vi "controllerPIP.vi"(11 "error in (no error)":errorcluster) -> (4 "FIXTURE_SETUP-1":string, 6 "POWER_UP-5, 6":string, 8 "RESISTANCE-15":string, 10 "INCLINE-14":string, 15 "error out":errorcluster)   [LabVIEW 2018]
uses:
  Global_1259.vi
panel:
  out "MTA":bool
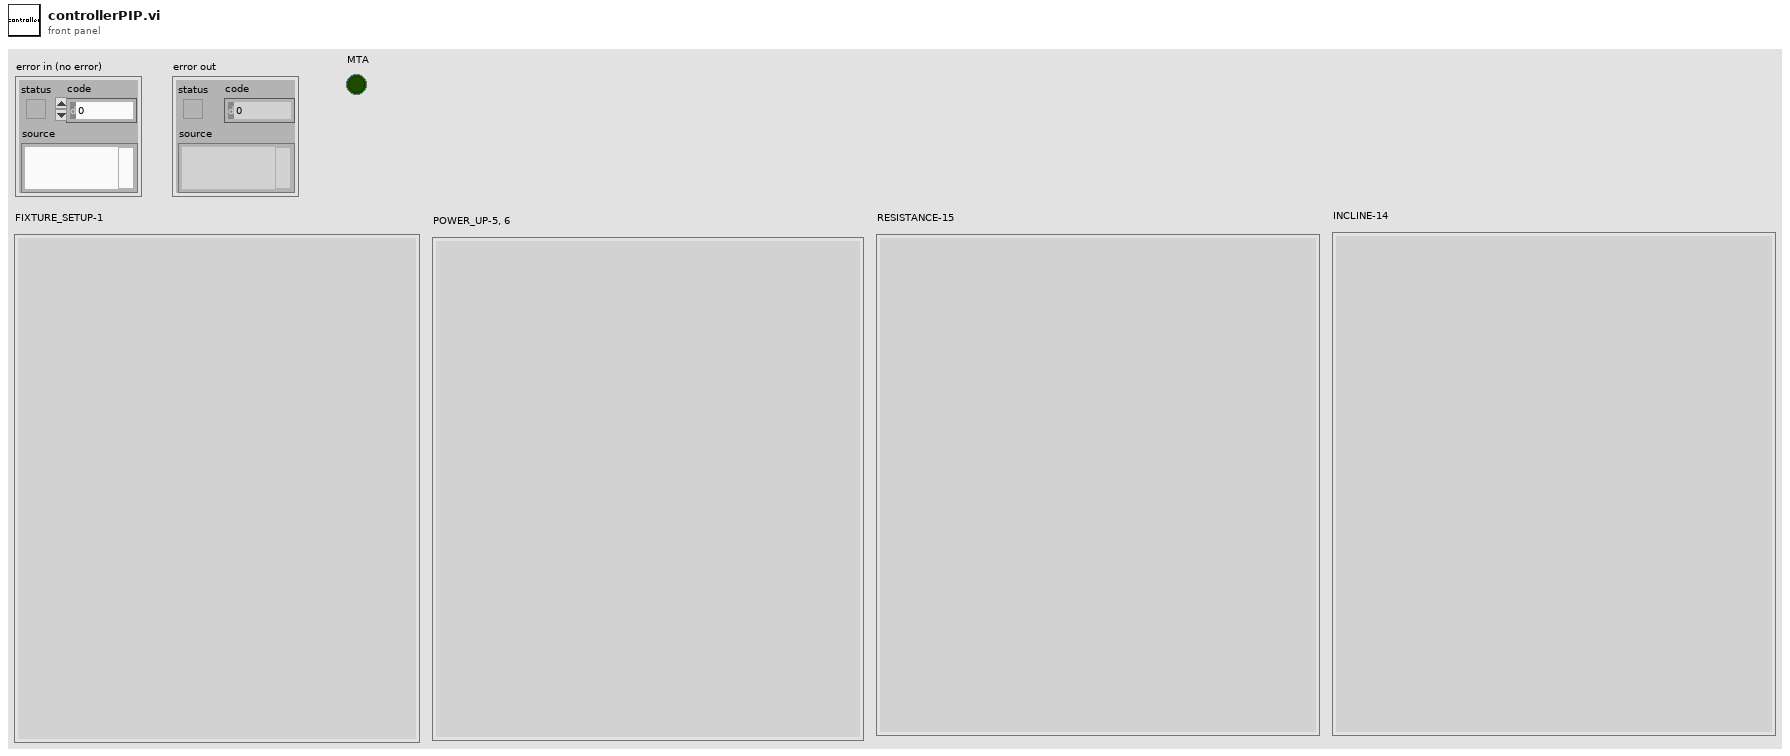
[diagram p1: front panel]
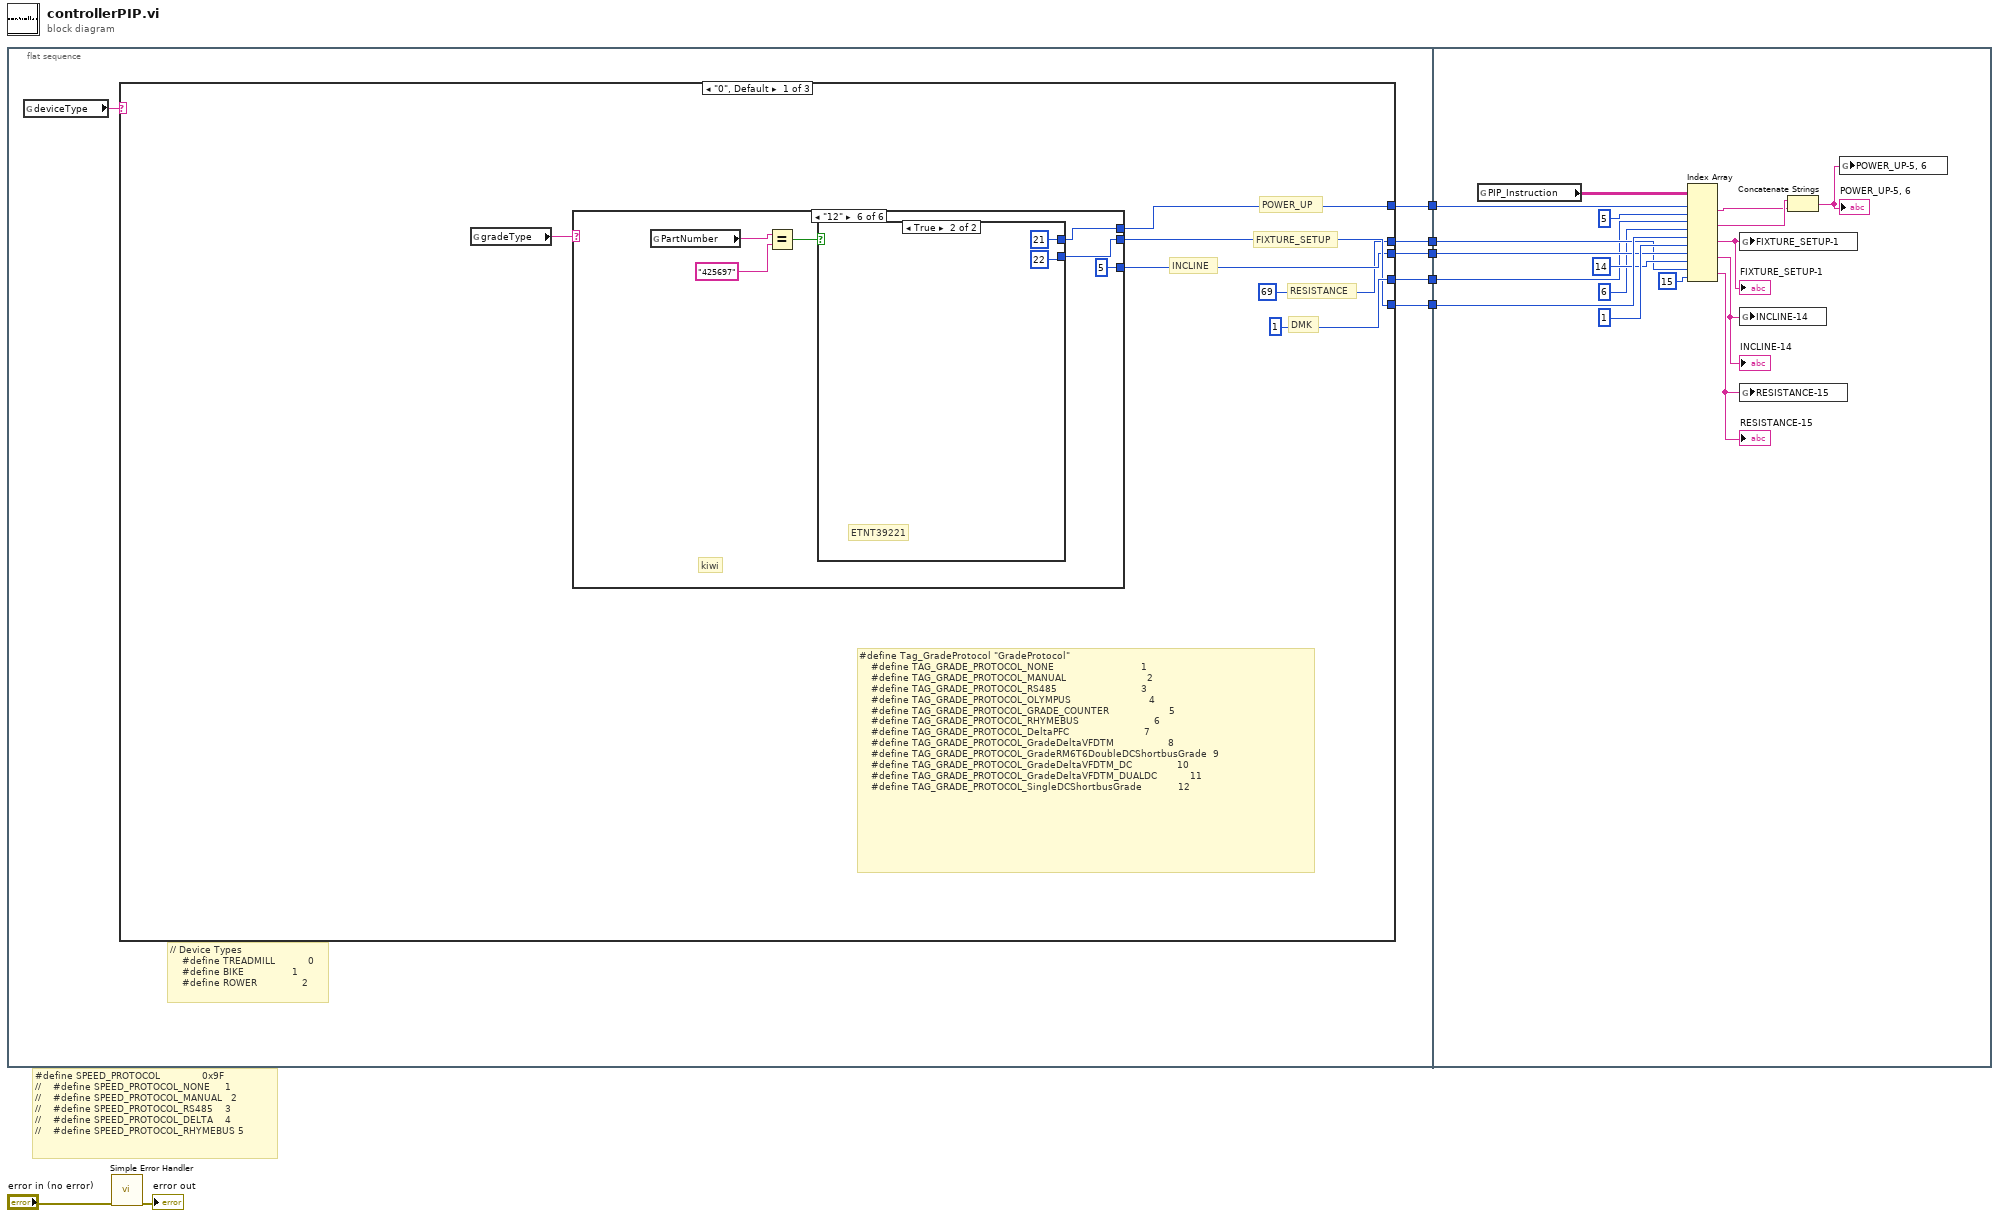
[diagram p0: block diagram]
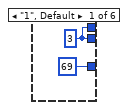
[diagram p2: hidden frame]
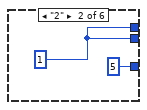
[diagram p3: hidden frame]
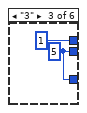
[diagram p4: hidden frame]
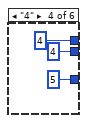
[diagram p5: hidden frame]
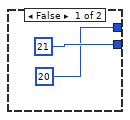
[diagram p7: hidden frame]
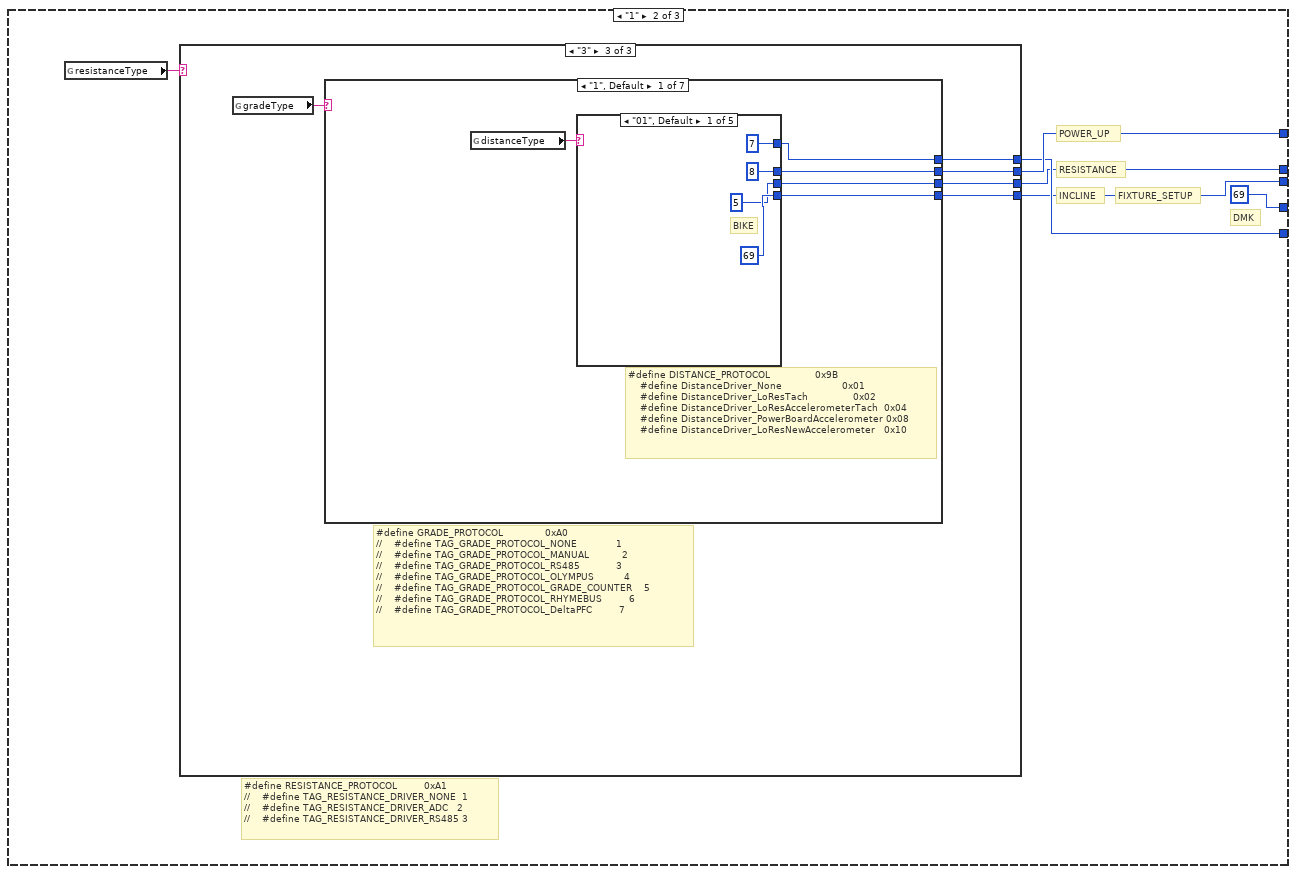
[diagram p8: hidden frame]
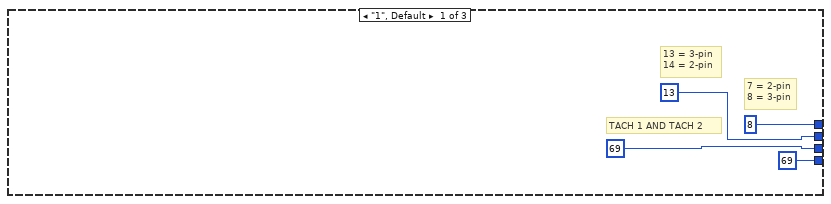
[diagram p9: hidden frame]
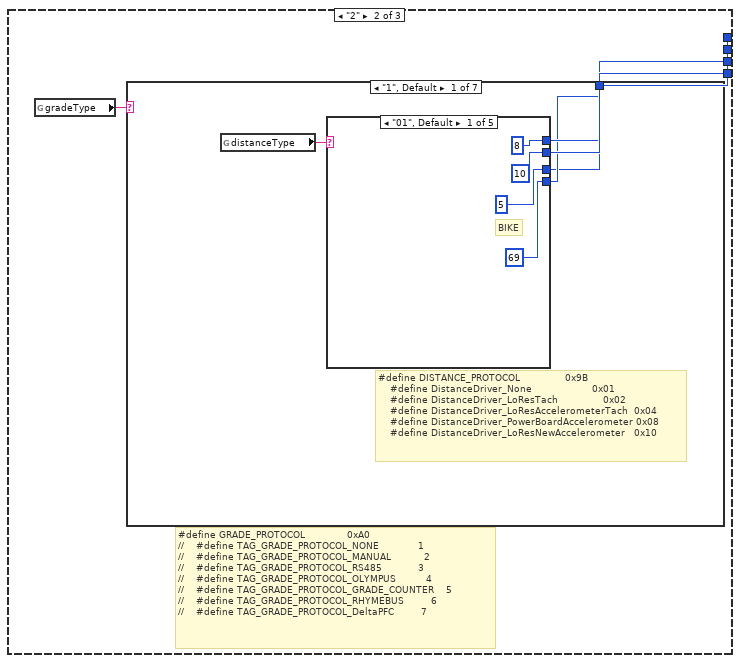
[diagram p10: hidden frame]
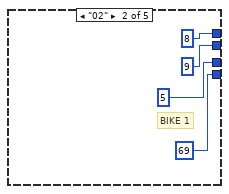
[diagram p11: hidden frame]
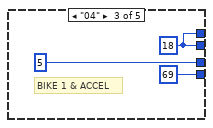
[diagram p12: hidden frame]
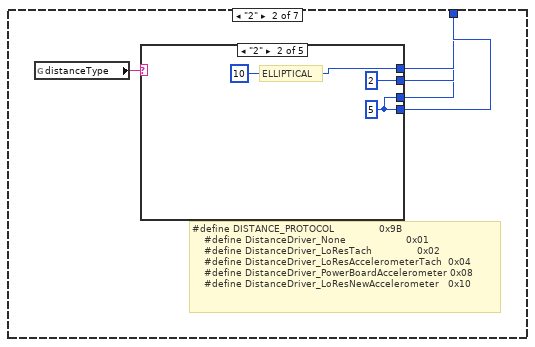
[diagram p15: hidden frame]
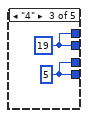
[diagram p17: hidden frame]
diagram:
  # "#define SPEED_PROTOCOL              0x9F\n//    #define SPEED_PROTOCOL_NONE     1\n//    #define SPEED_PROTOCOL_MANUAL   2\n//    #define SPEED_PROTOCOL_RS485    3\n//    #define SPEED_PROTOCOL_DELTA    4\n//    #define SPEED_PROTOCOL_RHYMEBUS 5"
  n1 = flat-sequence {
    tunnel: [w12] -> w7
    tunnel: [w11] -> w6
    tunnel: [w10] -> w5
    tunnel: [w9] -> w2
    tunnel: [w8] -> w1
    tunnel: w7 -> [w161]
    tunnel: w6 -> [w147]
    tunnel: w5 -> [w151]
    tunnel: w2 -> [w158]
    tunnel: w1 -> [w155]
    frame #0 {
      # "// Device Types\n    #define TREADMILL           0\n    #define BIKE                1\n    #define ROWER               2"
      n2 = global read "Global_1259.vi" "deviceType"() -> (w13:string)
      n3 = case shown="\"0\", Default" w13 {
        tunnel: [w17 w42 w116] -> w12
        tunnel: [1 69 w117] -> w11
        tunnel: [w14 w43 w114] -> w10
        tunnel: [w16 w41 w117] -> w9
        tunnel: [69 w40 w115] -> w8
        frame "0", Default {
          # "POWER_UP"
          # "RESISTANCE"
          # "#define Tag_GradeProtocol \"GradeProtocol\"\n    #define TAG_GRADE_PROTOCOL_NONE                             1\n    #define TAG_GRADE_PROTOCOL_MANUAL                           2\n    #define TAG_GRADE_PROTOCOL_RS485                            3\n    #define TAG_GRADE_PROTOCOL_OLYMPUS                          4\n    #define TAG_GRADE_PROTOCOL_GRADE_COUNTER                    5\n    #define TAG_GRADE_PROTOCOL_RHYMEBUS                         6\n    #define TAG_GRADE_PROTOCOL_DeltaPFC                         7\n    #define TAG_GRADE_PROTOCOL_GradeDeltaVFDTM                  8\n    #define TAG_GRADE_PROTOCOL_GradeRM6T6DoubleDCShortbusGrade  9\n    #define TAG_GRADE_PROTOCOL_GradeDeltaVFDTM_DC               10\n    #define TAG_GRADE_PROTOCOL_GradeDeltaVFDTM_DUALDC           11  \n    #define TAG_GRADE_PROTOCOL_SingleDCShortbusGrade            12"
          # "INCLINE"
          # "FIXTURE_SETUP"
          # "DMK"
          n4 = global read "Global_1259.vi" "gradeType"() -> (w19:string)
          n5 = case shown="\"12\"" w19 {
            tunnel: [w20 w22 w24 4 ("t") _ w32] -> w17
            tunnel: [69 ("t") 5 ("t") w24 5 ("t") _ 5 ("t")] -> w16
            tunnel: [w20 w22 1 ("t") 4 ("t") _ w31] -> w14
            frame "1", Default {
              w20 = 3 ("t")
            }
            frame "2" {
              w22 = 1 ("t")
            }
            frame "3" {
              w24 = 5 ("t")
            }
            frame "4" {
            }
            frame "5" {
            }
            frame "12" {
              # "kiwi"
              n6 = global read "Global_1259.vi" "PartNumber"() -> (w29:string)
              n7 = Equal?(x=w29, y="425697" ("x")) -> (x = y?=w33:bool)
              n8 = case shown="True" w33 {
                tunnel: [21 ("t") 22 ("t")] -> w32
                tunnel: [20 ("t") 21 ("t")] -> w31
                frame False {
                }
                frame True {
                  # "ETNT39221"
                }
              }
            }
          }
        }
        frame "1" {
          # "#define RESISTANCE_PROTOCOL         0xA1\n//    #define TAG_RESISTANCE_DRIVER_NONE  1\n//    #define TAG_RESISTANCE_DRIVER_ADC   2\n//    #define TAG_RESISTANCE_DRIVER_RS485 3"
          # "POWER_UP"
          # "DMK"
          # "FIXTURE_SETUP"
          # "INCLINE"
          # "RESISTANCE"
          n9 = global read "Global_1259.vi" "resistanceType"() -> (w39:string)
          n10 = case shown="\"3\"" w39 {
            tunnel: [13 w52 w80] -> w43
            tunnel: [8 w51 w81] -> w42
            tunnel: [69 w50 w82] -> w41
            tunnel: [69 w49 w83] -> w40
            frame "1", Default {
              # "TACH 1 AND TACH 2"
              # "7 = 2-pin\n8 = 3-pin"
              # "13 = 3-pin\n14 = 2-pin"
            }
            frame "2" {
              # "#define GRADE_PROTOCOL              0xA0\n//    #define TAG_GRADE_PROTOCOL_NONE             1\n//    #define TAG_GRADE_PROTOCOL_MANUAL           2\n//    #define TAG_GRADE_PROTOCOL_RS485            3\n//    #define TAG_GRADE_PROTOCOL_OLYMPUS          4\n//    #define TAG_GRADE_PROTOCOL_GRADE_COUNTER    5\n//    #define TAG_GRADE_PROTOCOL_RHYMEBUS         6\n//    #define TAG_GRADE_PROTOCOL_DeltaPFC         7"
              n11 = global read "Global_1259.vi" "gradeType"() -> (w53:string)
              n12 = case shown="\"1\", Default" w53 {
                tunnel: [w58 w71 _ _ _ _ _] -> w52
                tunnel: [w57 w72 _ _ _ _ _] -> w51
                tunnel: [w56 w73 _ _ _ _ _] -> w50
                tunnel: [w55 w70 _ _ _ _ _] -> w49
                frame "1", Default {
                  # "#define DISTANCE_PROTOCOL               0x9B\n    #define DistanceDriver_None                    0x01\n    #define DistanceDriver_LoResTach               0x02\n    #define DistanceDriver_LoResAccelerometerTach  0x04\n    #define DistanceDriver_PowerBoardAccelerometer 0x08\n    #define DistanceDriver_LoResNewAccelerometer   0x10"
                  n13 = global read "Global_1259.vi" "distanceType"() -> (w54:string)
                  n14 = case shown="\"01\", Default" w54 {
                    tunnel: [10 9 w69 _ _] -> w58
                    tunnel: [8 8 w69 _ _] -> w57
                    tunnel: [69 69 69 _ _] -> w56
                    tunnel: [5 5 5 _ _] -> w55
                    frame "01", Default {
                      # "BIKE"
                    }
                    frame "02" {
                      # "BIKE 1"
                    }
                    frame "04" {
                      w69 = 18
                      # "BIKE 1 & ACCEL"
                    }
                    frame "08" {
                    }
                    frame "10" {
                    }
                  }
                }
                frame "2" {
                  # "#define DISTANCE_PROTOCOL               0x9B\n    #define DistanceDriver_None                    0x01\n    #define DistanceDriver_LoResTach               0x02\n    #define DistanceDriver_LoResAccelerometerTach  0x04\n    #define DistanceDriver_PowerBoardAccelerometer 0x08\n    #define DistanceDriver_LoResNewAccelerometer   0x10"
                  n15 = global read "Global_1259.vi" "distanceType"() -> (w74:string)
                  n16 = case shown="\"2\"" w74 {
                    tunnel: [_ w75 w78 _ _] -> w73
                    tunnel: [_ 10 w79 _ _] -> w72
                    tunnel: [_ 2 w79 _ _] -> w71
                    tunnel: [_ w75 w78 _ _] -> w70
                    frame "1", Default {
                    }
                    frame "2" {
                      w75 = 5
                      # "ELLIPTICAL"
                    }
                    frame "4" {
                      w78 = 5
                      w79 = 19
                    }
                    frame "8" {
                    }
                    frame "10" {
                    }
                  }
                }
                frame "3" {
                }
                frame "4" {
                }
                frame "5" {
                }
                frame "6" {
                }
                frame "7" {
                }
              }
            }
            frame "3" {
              # "#define GRADE_PROTOCOL              0xA0\n//    #define TAG_GRADE_PROTOCOL_NONE             1\n//    #define TAG_GRADE_PROTOCOL_MANUAL           2\n//    #define TAG_GRADE_PROTOCOL_RS485            3\n//    #define TAG_GRADE_PROTOCOL_OLYMPUS          4\n//    #define TAG_GRADE_PROTOCOL_GRADE_COUNTER    5\n//    #define TAG_GRADE_PROTOCOL_RHYMEBUS         6\n//    #define TAG_GRADE_PROTOCOL_DeltaPFC         7"
              n17 = global read "Global_1259.vi" "gradeType"() -> (w84:string)
              n18 = case shown="\"1\", Default" w84 {
                tunnel: [w89 w102 3 _ _ _ _] -> w80
                tunnel: [w88 w103 11 _ _ _ _] -> w81
                tunnel: [w87 w104 w111 _ _ _ _] -> w82
                tunnel: [w86 w101 w111 _ _ _ _] -> w83
                frame "1", Default {
                  # "#define DISTANCE_PROTOCOL               0x9B\n    #define DistanceDriver_None                    0x01\n    #define DistanceDriver_LoResTach               0x02\n    #define DistanceDriver_LoResAccelerometerTach  0x04\n    #define DistanceDriver_PowerBoardAccelerometer 0x08\n    #define DistanceDriver_LoResNewAccelerometer   0x10"
                  n19 = global read "Global_1259.vi" "distanceType"() -> (w85:string)
                  n20 = case shown="\"01\", Default" w85 {
                    tunnel: [8 9 w100 _ _] -> w89
                    tunnel: [7 8 w100 _ _] -> w88
                    tunnel: [69 69 69 _ _] -> w87
                    tunnel: [5 5 5 _ _] -> w86
                    frame "01", Default {
                      # "BIKE"
                    }
                    frame "02" {
                      # "BIKE 1"
                    }
                    frame "04" {
                      w100 = 18
                      # "BIKE 1 & RS485"
                    }
                    frame "08" {
                    }
                    frame "10" {
                    }
                  }
                }
                frame "2" {
                  # "#define DISTANCE_PROTOCOL               0x9B\n    #define DistanceDriver_None                    0x01\n    #define DistanceDriver_LoResTach               0x02\n    #define DistanceDriver_LoResAccelerometerTach  0x04\n    #define DistanceDriver_PowerBoardAccelerometer 0x08\n    #define DistanceDriver_LoResNewAccelerometer   0x10"
                  n21 = global read "Global_1259.vi" "distanceType"() -> (w105:string)
                  n22 = case shown="\"04\"" w105 {
                    tunnel: [_ w106 w109 _ _] -> w104
                    tunnel: [_ 10 w110 _ _] -> w103
                    tunnel: [_ 2 w110 _ _] -> w102
                    tunnel: [_ w106 w109 _ _] -> w101
                    frame "01", Default {
                    }
                    frame "02" {
                      w106 = 5
                      # "ELLIPTICAL"
                    }
                    frame "04" {
                      w109 = 5
                      w110 = 19
                      # "ELLIPTICAL AND ACCEL"
                    }
                    frame "08" {
                    }
                    frame "10" {
                    }
                  }
                }
                frame "3" {
                  w111 = 5
                  # "RS485"
                }
                frame "4" {
                }
                frame "5" {
                }
                frame "6" {
                }
                frame "7" {
                }
              }
            }
          }
        }
        frame "2" {
          w117 = 69
          # "POWER_UP"
          # "DMK"
          # "FIXTURE_SETUP"
          # "INCLINE"
          # "RESISTANCE"
          n23 = global read "Global_1259.vi" "TABLET"() -> (w118:string)
          n24 = case shown="\"0\", Default" w118 {
            tunnel: [w119 20] -> w116
            tunnel: [w120 5] -> w115
            tunnel: [w121 16] -> w114
            frame "0", Default {
              # "BLE"
              n25 = while {
                tunnel: [w131] -> w122
                stop <- w130 stop-if-true
                n26 = global read "Global_1259.vi" "Part Name"() -> (w129:string)
                n27 = for {
                  tunnel: w129 -> [w143]
                  tunnel: string[] ["59147", "99147", "58118"] -> [w141] mode=indexing
                  tunnel: [w140] -> w132 mode=indexing
                  n28 = Match Pattern(string=w143, regular expression=w141) -> (match substring=w142:string)  [unwired: 1 in, 3 out]
                  n29 = Equal?(x=w141, y=w142) -> (x = y?=w140:bool)
                }
                n30 = while {
                  tunnel: w132 -> [w139]
                  tunnel: [w135] -> w130
                  tunnel: [w134] -> w131
                  i -> [w137]
                  stop <- w135 stop-if-true
                  n31 = Array Size(array=w139) -> (size(s)=w138:i32)
                  n32 = Equal?(x=w137, y=w138) -> (x = y?=w136:bool)
                  n33 = Index Array(array=w139, index=w137) -> (element=w134:bool)
                  n34 = Or(x=w134, y=w136) -> (x .or. y?=w135:bool)
                }
              }
              "MTA" <- w122
              n35 = case shown="False" w122 {
                tunnel: [20 10] -> w121
                tunnel: [1 1] -> w120
                tunnel: [21 8] -> w119
                frame False {
                  # "JST"
                }
                frame True {
                  # "MTA"
                }
              }
            }
            frame "1" {
              # "TABLET"
            }
          }
        }
      }
    }
    frame #1 {
      n36 = global read "Global_1259.vi" "PIP_Instruction"() -> (w150:string[][])
      n37 = Index Array(array=w150, index (row) #1=w151, index (col) #1=5 ("disabled index (col)"), index (row) #2=w147, index (col) #2=6 ("disabled index (col)"), index (row) #3=w161, index (col) #3=1 ("disabled index (col)"), index (row) #4=w158, index (col) #4=14 ("disabled index (col)"), index (row) #5=w155, index (col) #5=15 ("disabled index (col)")) -> (element #1=w148:string, element #2=w149:string, element #3=w160:string, element #4=w157:string, element #5=w154:string)
      "FIXTURE_SETUP-1" <- w160
      "INCLINE-14" <- w157
      "RESISTANCE-15" <- w154
      n38 = global write "Global_1259.vi" "FIXTURE_SETUP-1"(w160) -> ()
      n39 = global write "Global_1259.vi" "INCLINE-14"(w157) -> ()
      n40 = global write "Global_1259.vi" "RESISTANCE-15"(w154) -> ()
      n41 = Concatenate Strings(w149, w148) -> (w163:string)
      "POWER_UP-5, 6" <- w163
      n42 = global write "Global_1259.vi" "POWER_UP-5, 6"(w163) -> ()
    }
  }
  n43 = call <vilib>:"Simple Error Handler.vi"("error in (no error)"="error in (no error)") -> ("error out"=→"error out":errorcluster)  [unwired: 4 in, 4 out]
